vi "myRIO_BRig_Host_parse_dataTrial.vi"(11 "arrayIn_dataTrial":u16[][](array[numeric])) -> (2 "arrayOut_plotData":cluster{u8[], u8[]}[](array[cluster]))   [LabVIEW 2014]
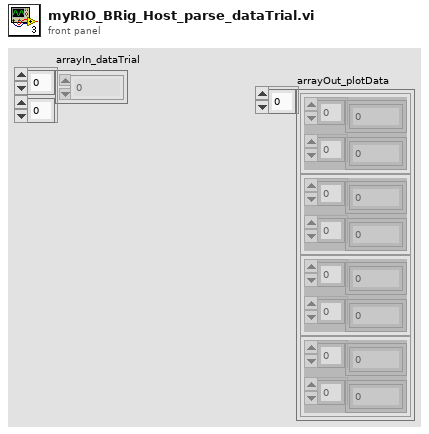
[diagram p1: front panel]
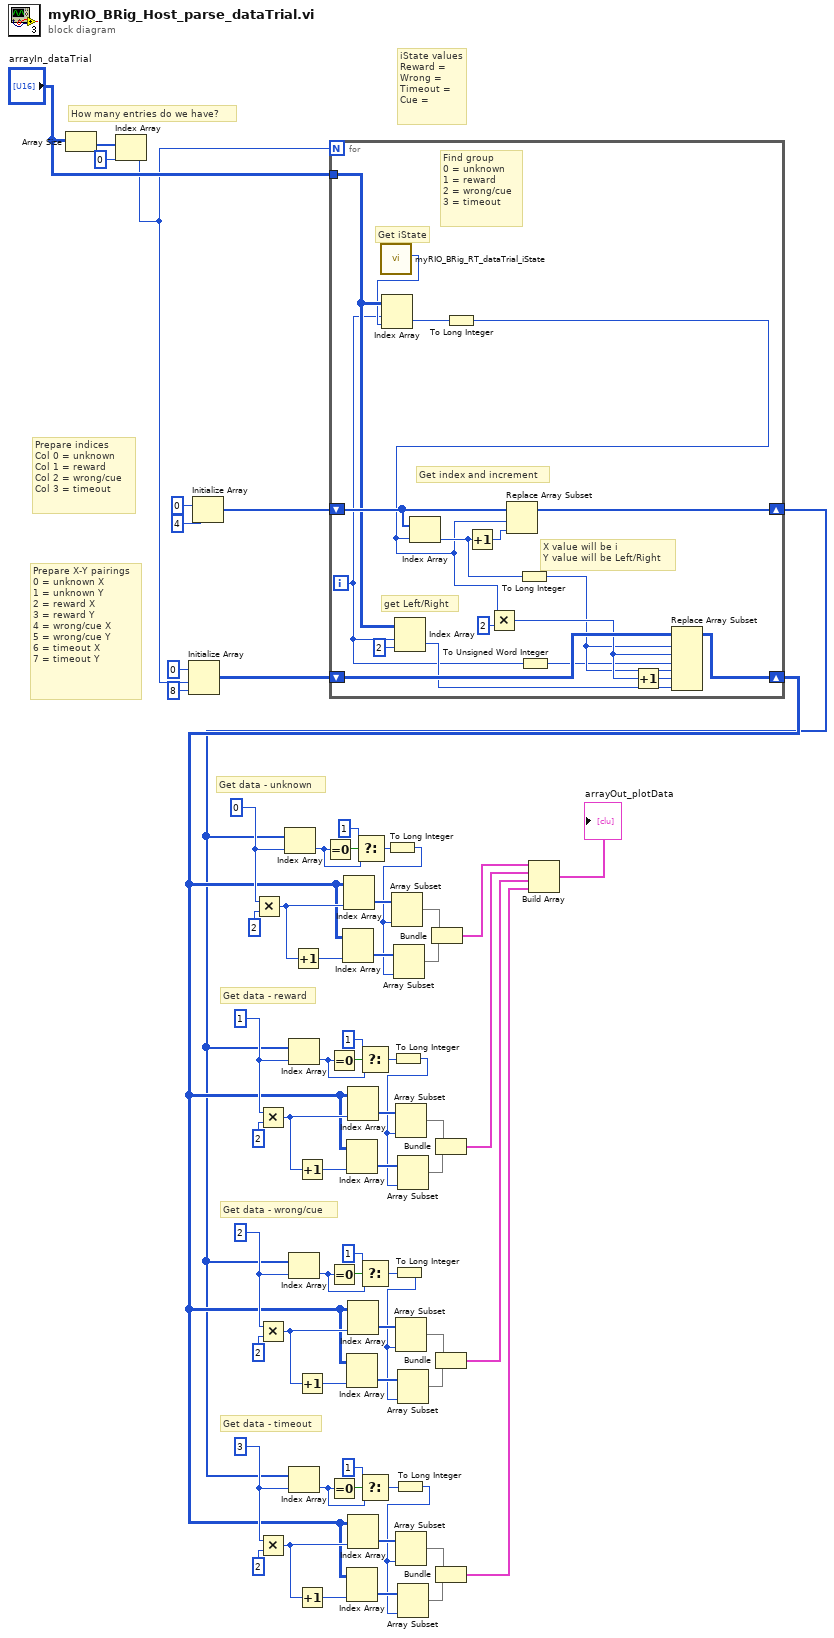
[diagram p0: block diagram]
diagram:
  w21 = 3 ("index")
  w32 = 2 ("index")
  w43 = 1 ("index")
  w54 = 0 ("index")
  # "Get data - timeout"
  # "Get data - wrong/cue"
  # "Get data - reward"
  # "Get data - unknown"
  # "Prepare X-Y pairings\n0 = unknown X\n1 = unknown Y\n2 = reward X\n3 = reward Y\n4 = wrong/cue X\n5 = wrong/cue Y\n6 = timeout X\n7 = timeout Y"
  # "Prepare indices\nCol 0 = unknown\nCol 1 = reward\nCol 2 = wrong/cue\nCol 3 = timeout"
  # "How many entries do we have?"
  # "iState values\nReward =\nWrong = \nTimeout = \nCue ="
  n1 = Array Size(array="arrayIn_dataTrial") -> (size(s)=w69:i32[])
  n2 = Index Array(array=w69, index=0) -> (element=w10:i32)
  n3 = Initialize Array(u16 0 ("element"), w10, 8 ("dimension size")) -> (w63:u16[][])
  n4 = Initialize Array(u16 0 ("element"), 4 ("dimension size")) -> (w62:u16[])
  n5 = Multiply(x=w54, y=2 ("index")) -> (x*y=w55:i32)
  n6 = Multiply(x=w43, y=2 ("index")) -> (x*y=w44:i32)
  n7 = Multiply(x=w32, y=2 ("index")) -> (x*y=w33:i32)
  n8 = Multiply(x=w21, y=2 ("index")) -> (x*y=w22:i32)
  n9 = Increment(x=w55) -> (x+1=w57:i32)
  n10 = Increment(x=w44) -> (x+1=w46:i32)
  n11 = Increment(x=w33) -> (x+1=w35:i32)
  n12 = Increment(x=w22) -> (x+1=w24:i32)
  n13 = for {
    N: w10 -> [_]
    shift-right: [w82] -> w16
    shift-left: w63 -> [w83]
    shift-right: [w86] -> w15
    shift-left: w62 -> [w87]
    tunnel: "arrayIn_dataTrial" -> [w77]
    i -> [w73]
    # "get Left/Right"
    # "X value will be i\nY value will be Left/Right"
    # "Get index and increment"
    # "Find group\n0 = unknown\n1 = reward\n2 = wrong/cue\n3 = timeout"
    # "Get iState"
    n14 = call "myRIO_BRig_RT_dataTrial_iState.vi"() -> ("output_iState"=w76:i32)  [unwired: 11 in]
    n15 = Index Array(array=w77, index (row)=w73, index (col)=w76) -> (element=w71:u16)
    n16 = Index Array(array=w77, index (row)=w73, index (col)=2 ("disabled index (col)")) -> (element=w81:u16)
    n17 = To Long Integer(number=w71) -> (32bit integer=w70:i32)
    n18 = Index Array(array=w87, index=w70) -> (element=w75:u16)
    n19 = Increment(x=w75) -> (x+1=w85:u16)
    n20 = Multiply(x=w70, y=2) -> (x*y=w78:i32)
    n21 = Replace Array Subset(array=w87, new element=w85, index=w70) -> (w86:u16[])
    n22 = To Long Integer(number=w75) -> (32bit integer=w74:i32)
    n23 = To Unsigned Word Integer(number=w73) -> (unsigned 16bit integer=w72:u16)
    n24 = Increment(x=w78) -> (x+1=w79:i32)
    n25 = Replace Array Subset(array=w83, new element #1=w72, index (row) #1=w74, index (col) #1=w78, new element #2=w81, index (row) #2=w74, index (col) #2=w79) -> (w82:u16[][])
  }
  n26 = Index Array(array=w15, index=w54) -> (element=w59:u16)
  n27 = Index Array(array=w15, index=w43) -> (element=w48:u16)
  n28 = Index Array(array=w15, index=w32) -> (element=w37:u16)
  n29 = Index Array(array=w15, index=w21) -> (element=w26:u16)
  n30 = Equal To 0?(x=w59) -> (x = 0?=w60:bool)
  n31 = Equal To 0?(x=w48) -> (x = 0?=w49:bool)
  n32 = Equal To 0?(x=w37) -> (x = 0?=w38:bool)
  n33 = Equal To 0?(x=w26) -> (x = 0?=w27:bool)
  n34 = Index Array(array=w16, index (col)=w57) -> (element=w56:u16[])  [unwired: 1 in]
  n35 = Index Array(array=w16, index (col)=w55) -> (element=w52:u16[])  [unwired: 1 in]
  n36 = Index Array(array=w16, index (col)=w46) -> (element=w45:u16[])  [unwired: 1 in]
  n37 = Index Array(array=w16, index (col)=w35) -> (element=w34:u16[])  [unwired: 1 in]
  n38 = Index Array(array=w16, index (col)=w24) -> (element=w23:u16[])  [unwired: 1 in]
  n39 = Index Array(array=w16, index (col)=w44) -> (element=w41:u16[])  [unwired: 1 in]
  n40 = Index Array(array=w16, index (col)=w33) -> (element=w30:u16[])  [unwired: 1 in]
  n41 = Index Array(array=w16, index (col)=w22) -> (element=w19:u16[])  [unwired: 1 in]
  n42 = Select(t=u16 1, s=w60, f=w59) -> (s? t:f=w8:u16)
  n43 = Select(t=u16 1, s=w49, f=w48) -> (s? t:f=w6:u16)
  n44 = Select(t=u16 1, s=w38, f=w37) -> (s? t:f=w4:u16)
  n45 = Select(t=u16 1, s=w27, f=w26) -> (s? t:f=w2:u16)
  n46 = To Long Integer(number=w8) -> (32bit integer=w7:i32)
  n47 = Array Subset(array=w52, length=w7) -> (w51:u16[])  [unwired: 1 in]
  n48 = To Long Integer(number=w6) -> (32bit integer=w5:i32)
  n49 = Array Subset(array=w56, length=w7) -> (w50:u16[])  [unwired: 1 in]
  n50 = To Long Integer(number=w4) -> (32bit integer=w3:i32)
  n51 = To Long Integer(number=w2) -> (32bit integer=w1:i32)
  n52 = Array Subset(array=w41, length=w5) -> (w40:u16[])  [unwired: 1 in]
  n53 = Array Subset(array=w30, length=w3) -> (w29:u16[])  [unwired: 1 in]
  n54 = Array Subset(array=w19, length=w1) -> (w18:u16[])  [unwired: 1 in]
  n55 = Array Subset(array=w45, length=w5) -> (w39:u16[])  [unwired: 1 in]
  n56 = Array Subset(array=w34, length=w3) -> (w28:u16[])  [unwired: 1 in]
  n57 = Array Subset(array=w23, length=w1) -> (w17:u16[])  [unwired: 1 in]
  n58 = Bundle(w51, w50) -> (w14:cluster{u16[], u16[]})  [unwired: 1 in]
  n59 = Bundle(w40, w39) -> (w13:cluster{u16[], u16[]})  [unwired: 1 in]
  n60 = Bundle(w29, w28) -> (w12:cluster{u16[], u16[]})  [unwired: 1 in]
  n61 = Bundle(w18, w17) -> (w11:cluster{u16[], u16[]})  [unwired: 1 in]
  n62 = Build Array(w14, w13, w12, w11) -> (→"arrayOut_plotData":cluster{u16[], u16[]}[])
